vi "Read Instrument Parameter(DMM).vi"(8 "error in (no error)":errorcluster) -> (0 "error out":errorcluster, 3 "DMM":T1)   [LabVIEW 2019, in "Unit Test Engine Tools.lvlib"]
uses:
  Unit Test Engine Tools.lvlib
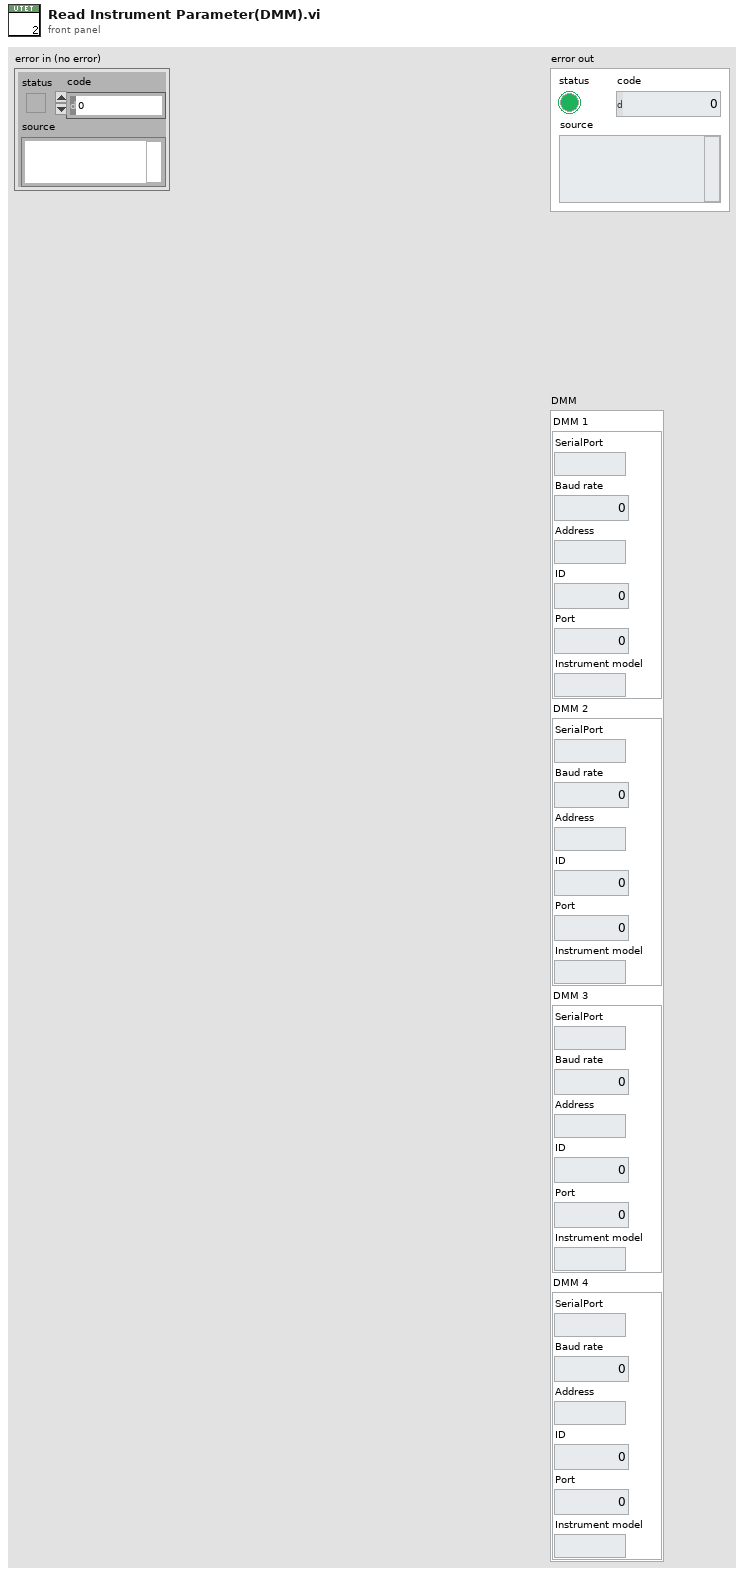
[diagram p1: front panel]
types:
  T1 = cluster{"DMM 1":cluster{"SerialPort":string, "Baud rate":i32, "Address":string, "ID":i32, "Port":i32, "Instrument model":string}, "DMM 2":cluster{"SerialPort":string, "Baud rate":i32, "Address":string, "ID":i32, "Port":i32, "Instrument model":string}, "DMM 3":cluster{"SerialPort":string, "Baud rate":i32, "Address":string, "ID":i32, "Port":i32, "Instrument model":string}, "DMM 4":cluster{"SerialPort":string, "Baud rate":i32, "Address":string, "ID":i32, "Port":i32, "Instrument model":string}}
  T2 = cluster{"LIN":cluster{"LIN 1":cluster{"Instrument model":string, "Port":string, "Baud rate":i32, "ID":i32, "Terminal":bool}, "LIN 2":cluster{"Instrument model":string, "Port":string, "Baud rate":i32, "ID":i32, "Terminal":bool}, "LIN 3":cluster{"Instrument model":string, "Port":string, "Baud rate":i32, "ID":i32, "Terminal":bool}, "LIN 4":cluster{"Instrument model":string, "Port":string, "Baud rate":i32, "ID":i32, "Terminal":bool}}, "Digital IO":cluster{"Digital IO 1":cluster{"SerialPort":string, "Baud rate":i32, "Address":string, "ID":i32, "Port":i32, "Instrument model":string}, "Digital IO 2":cluster{"SerialPort":string, "Baud rate":i32, "Address":string, "ID":i32, "Port":i32, "Instrument model":string}, "Digital IO 3":cluster{"SerialPort":string, "Baud rate":i32, "Address":string, "ID":i32, "Port":i32, "Instrument model":string}, "Digital IO 4":cluster{"SerialPort":string, "Baud rate":i32, "Address":string, "ID":i32, "Port":i32, "Instrument model":string}}, "DMM":cluster{"DMM 1":cluster{"SerialPort":string, "Baud rate":i32, "Address":string, "ID":i32, "Port":i32, "Instrument model":string}, "DMM 2":cluster{"SerialPort":string, "Baud rate":i32, "Address":string, "ID":i32, "Port":i32, "Instrument model":string}, "DMM 3":cluster{"SerialPort":string, "Baud rate":i32, "Address":string, "ID":i32, "Port":i32, "Instrument model":string}, "DMM 4":cluster{"SerialPort":string, "Baud rate":i32, "Address":string, "ID":i32, "Port":i32, "Instrument model":string}}, "Oscilloscope":cluster{"Oscilloscope 1":cluster{"SerialPort":string, "Baud rate":i32, "Address":string, "ID":i32, "Port":i32, "Instrument model":string}, "Oscilloscope 2":cluster{"SerialPort":string, "Baud rate":i32, "Address":string, "ID":i32, "Port":i32, "Instrument model":string}, "Oscilloscope 3":cluster{"SerialPort":string, "Baud rate":i32, "Address":string, "ID":i32, "Port":i32, "Instrument model":string}, "Oscilloscope 4":cluster{"SerialPort":string, "Baud rate":i32, "Address":string, "ID":i32, "Port":i32, "Instrument model":string}}, "PLC":cluster{"PLC 1":cluster{"SerialPort":string, "Baud rate":i32, "Address":string, "ID":i32, "Port":i32, "Instrument model":string}}, "ElectronicLoad":cluster{"ElectronicLoad 1":cluster{"SerialPort":string, "Baud rate":i32, "Address":string, "ID":i32, "Port":i32, "Instrument model":string}, "ElectronicLoad 2":cluster{"SerialPort":string, "Baud rate":i32, "Address":string, "ID":i32, "Port":i32, "Instrument model":string}, "ElectronicLoad 3":cluster{"SerialPort":string, "Baud rate":i32, "Address":string, "ID":i32, "Port":i32, "Instrument model":string}, "ElectronicLoad 4":cluster{"SerialPort":string, "Baud rate":i32, "Address":string, "ID":i32, "Port":i32, "Instrument model":string}}, "PowerSupply":cluster{"PowerSupply 1":cluster{"SerialPort":string, "Baud rate":i32, "Address":string, "ID":i32, "Port":i32, "Instrument model":string}, "PowerSupply 2":cluster{"SerialPort":string, "Baud rate":i32, "Address":string, "ID":i32, "Port":i32, "Instrument model":string}, "PowerSupply 3":cluster{"SerialPort":string, "Baud rate":i32, "Address":string, "ID":i32, "Port":i32, "Instrument model":string}, "PowerSupply 4":cluster{"SerialPort":string, "Baud rate":i32, "Address":string, "ID":i32, "Port":i32, "Instrument model":string}}, "CAN":cluster{"CAN 1":cluster{"Instrument model":string, "Port":string, "Baud rate":i32, "ID":i32, "Terminal":bool}, "CAN 2":cluster{"Instrument model":string, "Port":string, "Baud rate":i32, "ID":i32, "Terminal":bool}, "CAN 3":cluster{"Instrument model":string, "Port":string, "Baud rate":i32, "ID":i32, "Terminal":bool}, "CAN 4":cluster{"Instrument model":string, "Port":string, "Baud rate":i32, "ID":i32, "Terminal":bool}}, "Programming":cluster{"Programming 1":cluster{"Test Image":string, "Address":string, "Port":i32, "Instrument model":string, "Final Image":string}, "Programming 2":cluster{"Test Image":string, "Address":string, "Port":i32, "Instrument model":string, "Final Image":string}}, "Scanner":cluster{"Scanner 1":cluster{"SerialPort":string, "Baud rate":i32, "Address":string, "ID":i32, "Port":i32, "Instrument model":string}, "Scanner 2":cluster{"SerialPort":string, "Baud rate":i32, "Address":string, "ID":i32, "Port":i32, "Instrument model":string}, "Scanner 3":cluster{"SerialPort":string, "Baud rate":i32, "Address":string, "ID":i32, "Port":i32, "Instrument model":string}, "Scanner 4":cluster{"SerialPort":string, "Baud rate":i32, "Address":string, "ID":i32, "Port":i32, "Instrument model":string}}}
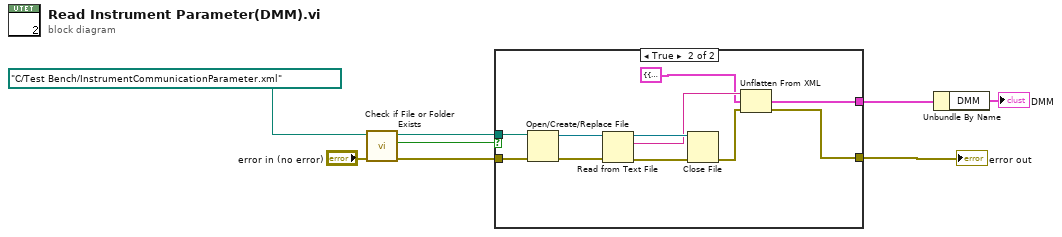
[diagram p0: block diagram]
diagram:
  n1 = call <vilib>:"Check if File or Folder Exists.vi"("error in (no error)"="error in (no error)", "path"=path "C:/Test Bench/InstrumentCommunicationParameter.xml") -> ("error out"=w7:errorcluster, "file or folder exists?"=w6:bool, "dup path"=w8:path)  [unwired: 7 in]
  n2 = case shown="True" w6 {
    tunnel: w8 -> [_ w20]
    tunnel: w7 -> [w9 w19]
    tunnel: [_ w13] -> w2
    tunnel: [w9 w11] -> w3
    frame False {
    }
    frame True {
      n3 = Open/Create/Replace File(file path (use dialog)=w20, error in=w19) -> (refnum out=w17:refnum<file>, error out=w18:errorcluster)  [unwired: 4 in, 1 out]
      n4 = Read from Text File(file (use dialog)=w17, error in=w18) -> (refnum out=w16:refnum<file>, text=w14:string, error out=w15:errorcluster)  [unwired: 2 in, 1 out]
      n5 = Close File(refnum=w16, error in=w15) -> (error out=w12:errorcluster)  [unwired: 1 out]
      n6 = Unflatten From XML(xml string=w14, type=T2 {"LIN"={"LIN 1"={"Instrument model"="", "Port"="", "Baud rate"=0, "ID"=0, "Terminal"=FALSE}, "LIN 2"={"Instrument model"="", "Port"="", "Baud rate"=0, "ID"=0, "Terminal"=FALSE}, "LIN 3"={"Instrument model"="", "Port"="", "Baud rate"=0, "ID"=0, "Terminal"=FALSE}, "LIN 4"={"Instrument model"="", "Port"="", "Baud rate"=0, "ID"=0, "Terminal"=FALSE}}, "Digital IO"={"Digital IO 1"={"SerialPort"="", "Baud rate"=0, "Address"="", "ID"=0, "Port"=0, "Instrument model"=""}, "Digital IO 2"={"SerialPort"="", "Baud rate"=0, "Address"="", "ID"=0, "Port"=0, "Instrument model"=""}, "Digital IO 3"={"SerialPort"="", "Baud rate"=0, "Address"="", "ID"=0, "Port"=0, "Instrument model"=""}, "Digital IO 4"={"SerialPort"="", "Baud rate"=0, "Address"="", "ID"=0, "Port"=0, "Instrument model"=""}}, "DMM"={"DMM 1"={"SerialPort"="", "Baud rate"=0, "Address"="", "ID"=0, "Port"=0, "Instrument model"=""}, "DMM 2"={"SerialPort"="", "Baud rate"=0, "Address"="", "ID"=0, "Port"=0, "Instrument model"=""}, "DMM 3"={"SerialPort"="", "Baud rate"=0, "Address"="", "ID"=0, "Port"=0, "Instrument model"=""}, "DMM 4"={"SerialPort"="", "Baud rate"=0, "Address"="", "ID"=0, "Port"=0, "Instrument model"=""}}, "Oscilloscope"={"Oscilloscope 1"={"SerialPort"="", "Baud rate"=0, "Address"="", "ID"=0, "Port"=0, "Instrument model"=""}, "Oscilloscope 2"={"SerialPort"="", "Baud rate"=0, "Address"="", "ID"=0, "Port"=0, "Instrument model"=""}, "Oscilloscope 3"={"SerialPort"="", "Baud rate"=0, "Address"="", "ID"=0, "Port"=0, "Instrument model"=""}, "Oscilloscope 4"={"SerialPort"="", "Baud rate"=0, "Address"="", "ID"=0, "Port"=0, "Instrument model"=""}}, "PLC"={"PLC 1"={"SerialPort"="", "Baud rate"=0, "Address"="", "ID"=0, "Port"=0, "Instrument model"=""}}, "ElectronicLoad"={"ElectronicLoad 1"={"SerialPort"="", "Baud rate"=0, "Address"="", "ID"=0, "Port"=0, "Instrument model"=""}, "ElectronicLoad 2"={"SerialPort"="", "Baud rate"=0, "Address"="", "ID"=0, "Port"=0, "Instrument model"=""}, "ElectronicLoad 3"={"SerialPort"="", "Baud rate"=0, "Address"="", "ID"=0, "Port"=0, "Instrument model"=""}, "ElectronicLoad 4"={"SerialPort"="", "Baud rate"=0, "Address"="", "ID"=0, "Port"=0, "Instrument model"=""}}, "PowerSupply"={"PowerSupply 1"={"SerialPort"="", "Baud rate"=0, "Address"="", "ID"=0, "Port"=0, "Instrument model"=""}, "PowerSupply 2"={"SerialPort"="", "Baud rate"=0, "Address"="", "ID"=0, "Port"=0, "Instrument model"=""}, "PowerSupply 3"={"SerialPort"="", "Baud rate"=0, "Address"="", "ID"=0, "Port"=0, "Instrument model"=""}, "PowerSupply 4"={"SerialPort"="", "Baud rate"=0, "Address"="", "ID"=0, "Port"=0, "Instrument model"=""}}, "CAN"={"CAN 1"={"Instrument model"="", "Port"="", "Baud rate"=0, "ID"=0, "Terminal"=FALSE}, "CAN 2"={"Instrument model"="", "Port"="", "Baud rate"=0, "ID"=0, "Terminal"=FALSE}, "CAN 3"={"Instrument model"="", "Port"="", "Baud rate"=0, "ID"=0, "Terminal"=FALSE}, "CAN 4"={"Instrument model"="", "Port"="", "Baud rate"=0, "ID"=0, "Terminal"=FALSE}}, "Programming"={"Programming 1"={"Test Image"="", "Address"="", "Port"=0, "Instrument model"="", "Final Image"=""}, "Programming 2"={"Test Image"="", "Address"="", "Port"=0, "Instrument model"="", "Final Image"=""}}, "Scanner"={"Scanner 1"={"SerialPort"="", "Baud rate"=0, "Address"="", "ID"=0, "Port"=0, "Instrument model"=""}, "Scanner 2"={"SerialPort"="", "Baud rate"=0, "Address"="", "ID"=0, "Port"=0, "Instrument model"=""}, "Scanner 3"={"SerialPort"="", "Baud rate"=0, "Address"="", "ID"=0, "Port"=0, "Instrument model"=""}, "Scanner 4"={"SerialPort"="", "Baud rate"=0, "Address"="", "ID"=0, "Port"=0, "Instrument model"=""}}} ("InstrumentCommunication"), error in (no error)=w12) -> (value=w13:T2, error out=w11:errorcluster)
    }
  }
  "error out" <- w3
  n7 = Unbundle By Name(w2) -> ("DMM"=→"DMM":T1)
